vi "Size of TPCANChannelInformation--constant.vi"() -> (3 "Size of TPCANChannelInformation":u32)   [LabVIEW 2018, in "PCANBasic.lvlib"]
doc: "Size of TPCANChannelInformation which describes an available PCAN channel\n\ntypedef struct tagTPCANChannelInformation\n{\n TPCANHandle channel_handle; // PCAN channel handle \n TPCANDevice device_type; // Kind of PCAN device\n BYTE controller_number; // CAN-Controller number\n DWORD device_features; // Device capabilities flag (see FEATURE_*)\n char device_name[MAX_LENGTH_HARDWARE_NAME]; // Device name\n DWORD device_id; // Device number \n DWORD channel_condition; // Availability status of a PCAN-Channel \n}TPCANChannelInformation;"
uses:
  PCANBasic.lvlib
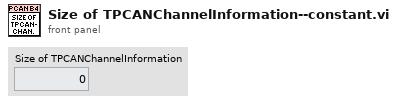
[diagram p1: front panel]
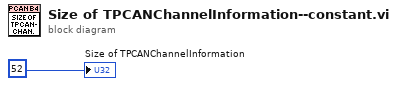
[diagram p0: block diagram]
diagram:
  "Size of TPCANChannelInformation" <- u32 52 ("x")
